vi "OMV_Initialize.vi"(6 "timeout":dbl=0.2 format="%#_13g", 9 "Port":string, 11 "Python":T1) -> (0 "error out":errorcluster, 2 "Version":string, 3 "Python":T1)   [LabVIEW 2020]
uses:
  PythonCtrl.ctl
  _subs/Processors.ctl
panel:
  out "Reply":string
  out "Tx for stopping code":string
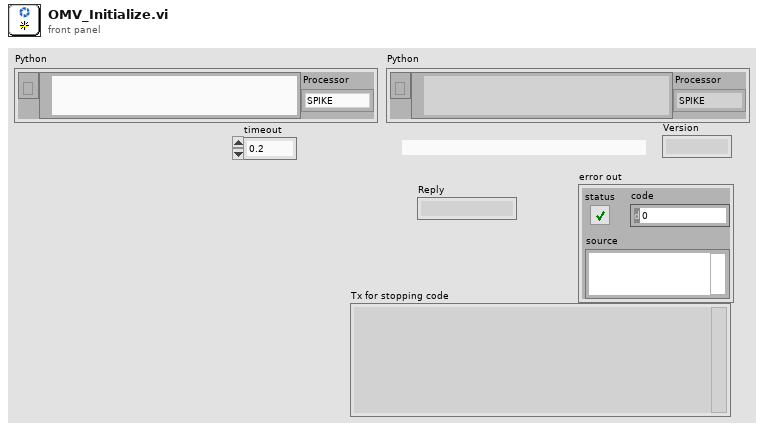
[diagram p1: front panel]
types:
  T1 = typedef "PythonCtrl.ctl" = cluster{"session":refnum<k35>, "PyPath":path, "Processor":T2}
  T2 = typedef "Processors.ctl" = enum16{"SPIKE", "Pi", "Pi_ssh", "OpenMV"}
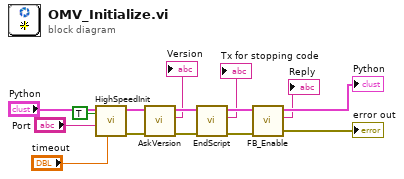
[diagram p0: block diagram]
diagram:
  n1 = call "HighSpeedInit.vi"("timeout"="timeout", "Port"="Port", "Fast"=TRUE, "Python"="Python") -> ("error out"=w11:errorcluster, "Python"=w12:T1)  [unwired: 6 in]
  n2 = call "AskVersion.vi"("error in"=w11, "Python"=w12) -> ("error out"=w14:errorcluster, "Version"=→"Version":string, "Python"=w15:T1)  [unwired: 7 in]
  n3 = call "EndScript.vi"("error in (no error)"=w14, "Python"=w15) -> ("error out"=w8:errorcluster, "Tx for stopping code"=→"Tx for stopping code":string, "Python"=w10:T1)  [unwired: 7 in]
  n4 = call "FB_Enable.vi"("error in"=w8, "Python"=w10) -> ("error out"=→"error out":errorcluster, "Reply"=→"Reply":string, "Python"=→"Python":T1)  [unwired: 7 in]
